vi "clear_line.vi"(11 "Array in":u8[][](array[numeric])) -> (1 "得分":u32, 2 "消除數":u8, 3 "Array out":u8[][](array[numeric]))   [LabVIEW 2024]
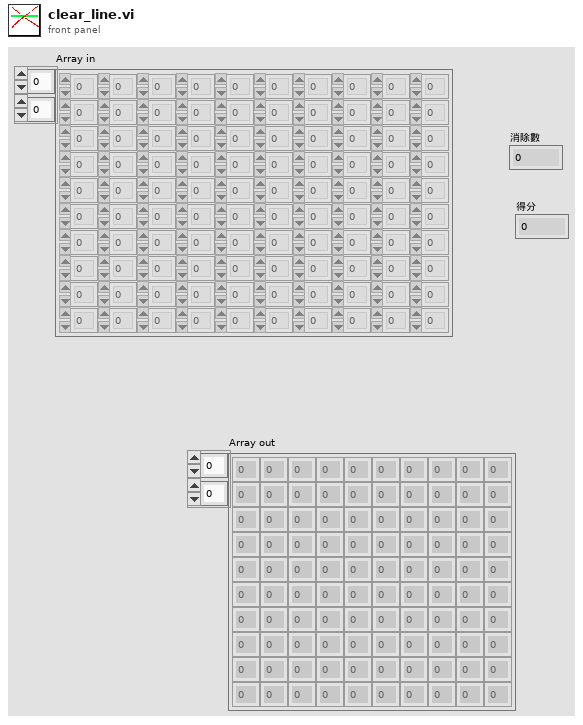
[diagram p1: front panel]
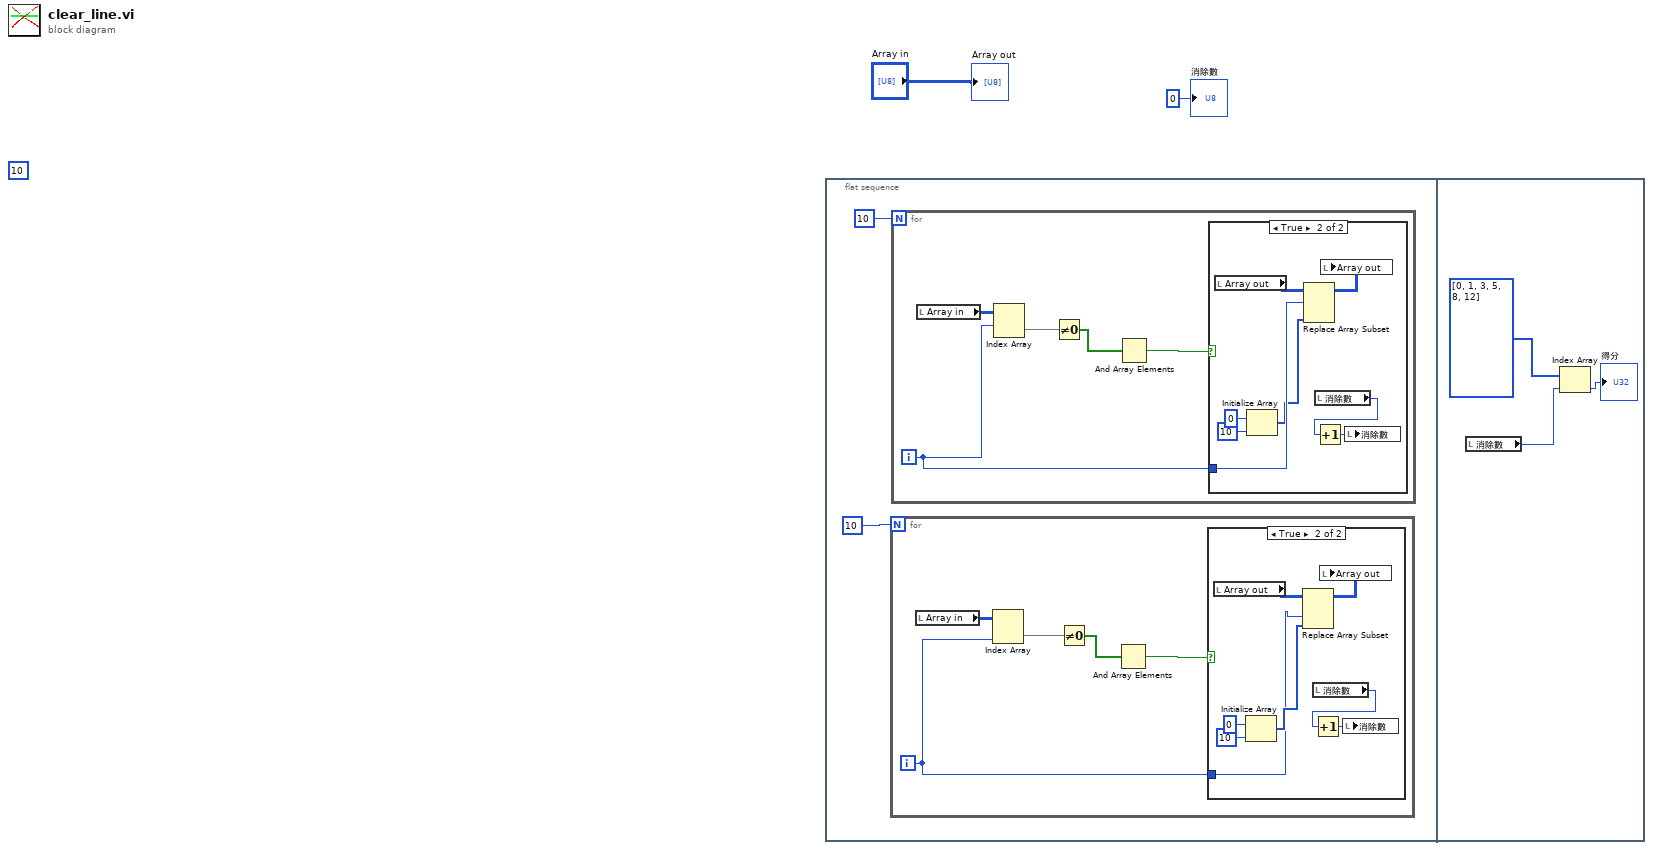
[diagram p0: block diagram]
diagram:
  (unwired) 10
  n1 = flat-sequence {
    frame #0 {
      n2 = for {
        N: 10 -> [_]
        i -> [w5]
        n3 = local read "Array in"() -> (w6:u8[][])
        n4 = Index Array(array=w6, index (col)=w5) -> (element=w9:u8[])  [unwired: 1 in]
        n5 = Not Equal To 0?(x=w9) -> (x != 0?=w7:bool[])
        n6 = And Array Elements(Boolean array=w7) -> (logical AND=w8:bool)
        n7 = case shown="True" w8 {
          tunnel: w5 -> [_ w12]
          frame False {
          }
          frame True {
            n8 = local read "Array out"() -> (w17:u8[][])
            n9 = Initialize Array(u8 0 ("element"), 10 ("dimension size")) -> (w13:u8[])
            n10 = Replace Array Subset(array=w17, new element=w13, index (col)=w12) -> (w16:u8[][])  [unwired: 1 in]
            n11 = local read "消除數"() -> (w10:u8)
            n12 = Increment(x=w10) -> (x+1=w11:u8)
            n13 = local write "Array out"(w16) -> ()
            n14 = local write "消除數"(w11) -> ()
          }
        }
      }
      n15 = for {
        N: 10 -> [_]
        i -> [w21]
        n16 = local read "Array in"() -> (w18:u8[][])
        n17 = Index Array(array=w18, index (row)=w21) -> (element=w22:u8[])  [unwired: 1 in]
        n18 = Not Equal To 0?(x=w22) -> (x != 0?=w19:bool[])
        n19 = And Array Elements(Boolean array=w19) -> (logical AND=w20:bool)
        n20 = case shown="True" w20 {
          tunnel: w21 -> [_ w29]
          frame False {
          }
          frame True {
            n21 = local read "Array out"() -> (w30:u8[][])
            n22 = Initialize Array(u8 0 ("element"), 10 ("dimension size")) -> (w25:u8[])
            n23 = Replace Array Subset(array=w30, new element=w25, index (row)=w29) -> (w28:u8[][])  [unwired: 1 in]
            n24 = local read "消除數"() -> (w23:u8)
            n25 = Increment(x=w23) -> (x+1=w24:u8)
            n26 = local write "Array out"(w28) -> ()
            n27 = local write "消除數"(w24) -> ()
          }
        }
      }
    }
    frame #1 {
      n28 = local read "消除數"() -> (w32:u8)
      n29 = Index Array(array=u32[] [0, 1, 3, 5, 8, 12], index=w32) -> (element=→"得分":u32)
    }
  }
  "Array out" <- "Array in"
  "消除數" <- u8 0 ("消除數")
